vi "event_message.vi"(4 "message":refnum<vi>, 5 "Event Data":cluster{"message":string}, 6 "Control Ref":refnum<k7>, 7 "Event Common Data":T1) -> ()   [LabVIEW 2010]
panel:
  out "error out":errorcluster
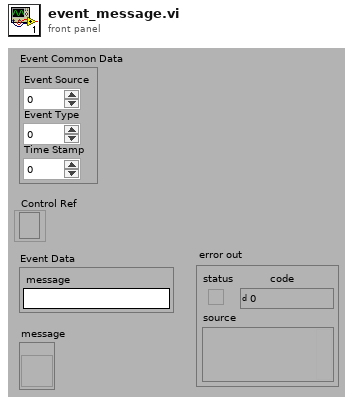
[diagram p1: front panel]
types:
  T1 = cluster{"Event Source":i32, "Event Type":u32, "Time Stamp":u32}
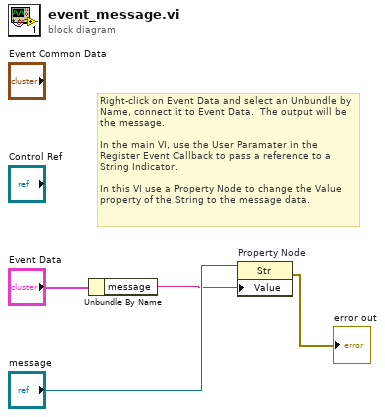
[diagram p0: block diagram]
diagram:
  # "Right-click on Event Data and select an Unbundle by Name, connect it to Event Data.  The output will be the message.\n\nIn the main VI, use the User Paramater in the Register Event Callback to pass a reference to a String Indicator.  \n\nIn this VI use a Property Node to change the Value property of the String to the message data."
  n1 = Unbundle By Name "Unbundle By Name"("Event Data") -> ("message"=w2:string)
  n2 = property on="Property Node" class="Str"(reference="message", "Value"=w2) -> (error out=→"error out":errorcluster)  [unwired: 1 in, 1 out]
